vi "Rohde & Schwarz VNA Read Status Bit.vi"(7 "Anritsu VNA":T1, 8 "error in (no error)":errorcluster, 11 "VISA Resource Name":refnum<visa-resource-name>) -> (0 "error out":errorcluster, 2 "Status Bit":bool, 3 "dup VISA Resource Name":refnum<visa-resource-name>)   [LabVIEW 2011]
doc: "This VI for the HP8753B Network Analyzer reads the status byte and the two event status registers. The two status registers are read out as regular output and will therefore clear anything already in the output queue."
uses:
  Anritsu/TypeDefs/Anritsu VNA Instrument Info.ctl
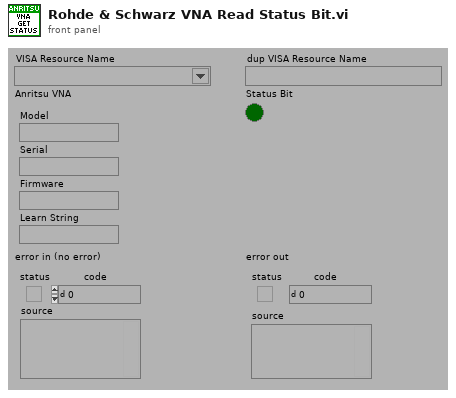
[diagram p1: front panel]
types:
  T1 = typedef "Anritsu VNA Instrument Info.ctl" = cluster{"Model":string, "Serial":string, "Firmware":string, "Learn String":string}
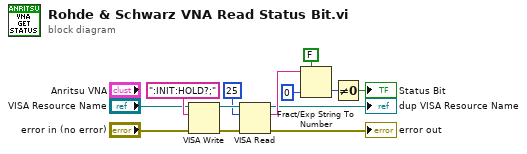
[diagram p0: block diagram]
diagram:
  n1 = VISA Write(VISA resource name="VISA Resource Name", write buffer=":INIT:HOLD?;", error in (no error)="error in (no error)") -> (VISA resource name out=w12:refnum<visa-resource-name>, error out=w13:errorcluster)  [unwired: 1 out]
  n2 = VISA Read(VISA resource name=w12, byte count=u32 25, error in (no error)=w13) -> (VISA resource name out=→"dup VISA Resource Name":refnum<visa-resource-name>, read buffer=w9:string, error out=→"error out":errorcluster)  [unwired: 1 out]
  n3 = Fract/Exp String To Number(use system decimal point (T)=FALSE, string=w9, default (0 dbl)=0 ("default (0 DBL)")) -> (number=w2:i32)  [unwired: 2 out]
  n4 = Not Equal To 0?(x=w2) -> (x != 0?=→"Status Bit":bool)
